vi "3.11-Graph Equation.vi"(1 "X":i32, 2 "Graph scale factor (b)":dbl, 3 "Where it hits 0 (z)":dbl, 4 "parabolic constant (c)":dbl) -> (0 "Y":dbl)   [LabVIEW 2010]
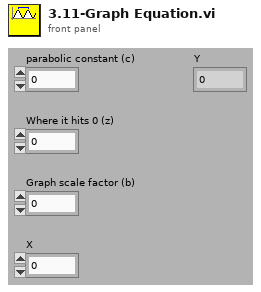
[diagram p1: front panel]
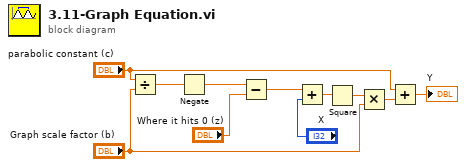
[diagram p0: block diagram]
diagram:
  n1 = Divide(x="parabolic constant (c)", y="Graph scale factor (b)") -> (x/y=w1:dbl)
  n2 = Negate(x=w1) -> (-x=w3:dbl)
  n3 = Subtract(x=w3, y="Where it hits 0 (z)") -> (x-y=w4:dbl)
  n4 = Add(x=w4, y="X") -> (x+y=w6:dbl)
  n5 = Square(x=w6) -> (x^2=w11:dbl)
  n6 = Multiply(x=w11, y="Graph scale factor (b)") -> (x*y=w8:dbl)
  n7 = Add(x="parabolic constant (c)", y=w8) -> (x+y=→"Y":dbl)
